vi "DAQ Multiple Uses of Task (Digital IO and Counter) - LV2012 NI Verified.vi"() -> ()   [LabVIEW 2015]
uses:
  <vilib>/DAQmx/read.llb/DAQmx Read (Counter DBL 1Chan 1Samp).vi
  <vilib>/DAQmx/write.llb/DAQmx Write (Digital 1D Bool NChan 1Samp 1Line).vi
  <vilib>/DAQmx/read.llb/DAQmx Read (Digital 1D Bool NChan 1Samp 1Line).vi
  <vilib>/DAQmx/create/channels.llb/DAQmx Create Channel (DI-Digital Input).vi
  <vilib>/DAQmx/create/channels.llb/DAQmx Create Channel (DO-Digital Output).vi
  <vilib>/DAQmx/create/channels.llb/DAQmx Create Channel (CI-Frequency).vi
  <vilib>/DAQmx/miscellaneous.llb/DAQmx Fill In Error Info.vi
panel:
  in  "stop":bool
  out "Counter In Freq":dbl format="%0.2f"
  out "Digital Input Data":bool[](array[boolean])
  in  "Digital Output Data":bool[](array[boolean])
  # "Overview: Demonstrates a simple VI of using the three parallel lines of the DAQ hardware \nRequirement: LabVIEW Full Development System\nInstructions:\n1. Run the VI"
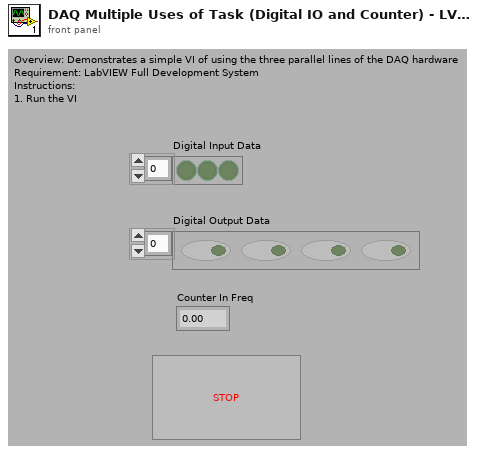
[diagram p1: front panel]
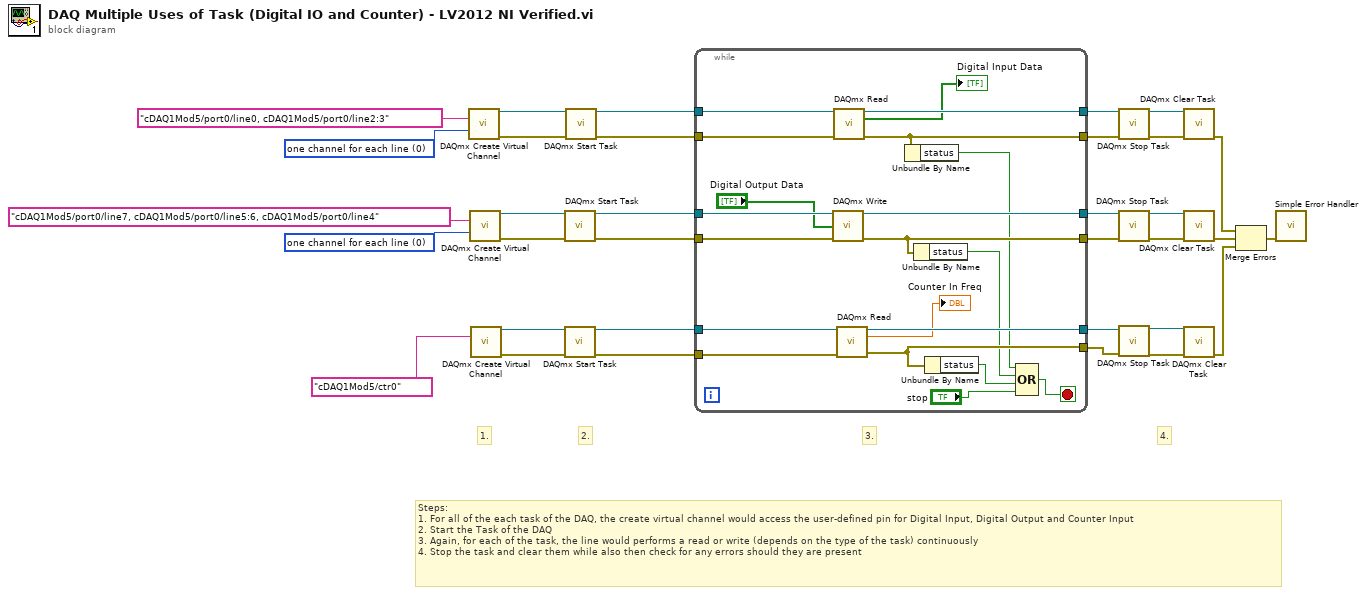
[diagram p0: block diagram]
diagram:
  w22 = 0 items=["one channel for each line", "one channel for all lines"] ("line grouping")
  w31 = 0 items=["one channel for each line", "one channel for all lines"] ("line grouping")
  # "Steps:\n1. For all of the each task of the DAQ, the create virtual channel would access the user-defined pin for Digital Input, Digital Output and Counter Input\n2. Start the Task of the DAQ\n3. Again, for each of the task, the line would performs a read or write (depends on the type of the task) continuously\n4. Stop the task and clear them while also then check for any errors should they are present"
  # "4."
  # "3."
  # "2."
  # "1."
  n1 = call-poly <vilib>:"DAQmx Create Virtual Channel.vi"("lines"=tag "cDAQ1Mod5/port0/line0, cDAQ1Mod5/port0/line2:3" ("Digital Input Lines"), "line grouping"=w22) -> ("task out"=w30:refnum<k21>, "error out"=w29:errorcluster)  [unwired: 3 in, 9 out]
  n2 = call-poly <vilib>:"DAQmx Create Virtual Channel.vi"("lines"=tag "cDAQ1Mod5/port0/line7, cDAQ1Mod5/port0/line5:6, cDAQ1Mod5/port0/line4" ("Digital Output Lines"), "line grouping"=w31) -> ("task out"=w26:refnum<k21>, "error out"=w25:errorcluster)  [unwired: 3 in, 9 out]
  n3 = call-poly <vilib>:"DAQmx Create Virtual Channel.vi"("counter"=tag "cDAQ1Mod5/ctr0" ("Counter Input Lines")) -> ("task out"=w18:refnum<k21>, "error out"=w19:errorcluster)  [unwired: 11 in, 2 out]
  n4 = call <vilib>:"DAQmx Start Task.vi"("task/channels in"=w26, "error in"=w25) -> ("task out"=w24:refnum<k21>, "error out"=w23:errorcluster)  [unwired: 12 out]
  n5 = call <vilib>:"DAQmx Start Task.vi"("task/channels in"=w18, "error in"=w19) -> ("task out"=w20:refnum<k21>, "error out"=w21:errorcluster)  [unwired: 12 out]
  n6 = call <vilib>:"DAQmx Start Task.vi"("task/channels in"=w30, "error in"=w29) -> ("task out"=w28:refnum<k21>, "error out"=w27:errorcluster)  [unwired: 12 out]
  n7 = while {
    tunnel: [w53] -> w12
    tunnel: [w40] -> w11
    tunnel: w28 -> [w52]
    tunnel: w27 -> [w51]
    tunnel: w24 -> [w50]
    tunnel: w23 -> [w49]
    tunnel: [w48] -> w16
    tunnel: [w41] -> w15
    tunnel: [w39] -> w7
    tunnel: [w45] -> w8
    tunnel: w21 -> [w44]
    tunnel: w20 -> [w43]
    stop <- w35 stop-if-true
    n8 = call-poly <vilib>:"DAQmx Write.vi"("task/channels in"=w50, "data"="Digital Output Data", "error in"=w49) -> ("task out"=w53:refnum<k21>, "error out"=w40:errorcluster)  [unwired: 1 in, 10 out]
    n9 = call-poly <vilib>:"DAQmx Read.vi"("task/channels in"=w52, "error in"=w51) -> ("task out"=w48:refnum<k21>, "data"=→"Digital Input Data":bool[], "error out"=w41:errorcluster)  [unwired: 1 in, 10 out]
    n10 = call-poly <vilib>:"DAQmx Read.vi"("task/channels in"=w43, "error in"=w44) -> ("task out"=w45:refnum<k21>, "data"=→"Counter In Freq":dbl, "error out"=w39:errorcluster)  [unwired: 11 out]
    n11 = Unbundle By Name(w41) -> ("status"=w38:bool)
    n12 = Unbundle By Name(w40) -> ("status"=w37:bool)
    n13 = Unbundle By Name(w39) -> ("status"=w36:bool)
    n14 = Compound Arithmetic op=OR(w38, w37, w36, "stop") -> (w35:bool)
  }
  n15 = call <vilib>:"DAQmx Stop Task.vi"("task/channels in"=w16, "error in"=w15) -> ("task out"=w14:refnum<k21>, "error out"=w13:errorcluster)  [unwired: 12 out]
  n16 = call <vilib>:"DAQmx Stop Task.vi"("task/channels in"=w12, "error in"=w11) -> ("task out"=w10:refnum<k21>, "error out"=w9:errorcluster)  [unwired: 12 out]
  n17 = call <vilib>:"DAQmx Stop Task.vi"("task/channels in"=w8, "error in"=w7) -> ("task out"=w6:refnum<k21>, "error out"=w5:errorcluster)  [unwired: 12 out]
  n18 = call <vilib>:"DAQmx Clear Task.vi"("task in"=w14, "error in"=w13) -> ("error out"=w4:errorcluster)  [unwired: 13 out]
  n19 = call <vilib>:"DAQmx Clear Task.vi"("task in"=w10, "error in"=w9) -> ("error out"=w3:errorcluster)  [unwired: 13 out]
  n20 = call <vilib>:"DAQmx Clear Task.vi"("task in"=w6, "error in"=w5) -> ("error out"=w2:errorcluster)  [unwired: 13 out]
  n21 = Merge Errors(w4, w3, w2) -> (w1:errorcluster)
  n22 = call <vilib>:"Simple Error Handler.vi"("error in (no error)"=w1) -> ()  [unwired: 4 in, 5 out]
